vi "Call Mass Compile CLI.vi"(8 "error in":errorcluster, 11 "Directory":path) -> (0 "error out":errorcluster)   [LabVIEW 2021, in "LV Scripting Utilities.lvlib"]
uses:
  LV Scripting Utilities.lvlib
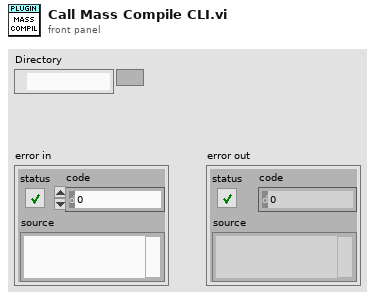
[diagram p1: front panel]
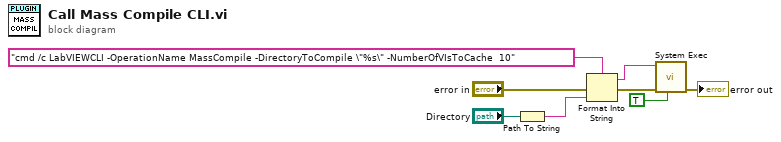
[diagram p0: block diagram]
diagram:
  n1 = Path To String(path="Directory") -> (string=w2:string)
  n2 = Format Into String(format string="cmd /c LabVIEWCLI -OperationName MassCompile -DirectoryToCompile \"%s\" -NumberOfVIsToCache  10" ("command line"), error in="error in", w2) -> (resulting string=w7:string, error out=w4:errorcluster)  [unwired: 1 in]
  n3 = call <vilib>:"System Exec.vi"("run minimized? (F)"=TRUE, "error in (no error)"=w4, "command line"=w7) -> ("error out"=→"error out":errorcluster)  [unwired: 5 in, 3 out]
